vi "AI0.vi"(8 "error in (no error)":errorcluster caption="错误输入（无错误）") -> (0 "error out":errorcluster caption="错误输出", 3 "Ai0波形":waveform(dbl)(graph))   [LabVIEW 2016]
uses:
  <vilib>/DAQmx/read.llb/DAQmx Read (Analog Wfm 1Chan NSamp).vi
  <vilib>/DAQmx/create/channels.llb/DAQmx Create Channel (AI-Voltage-Basic).vi
  <vilib>/DAQmx/configure/timing.llb/DAQmx Timing (Sample Clock).vi
  <vilib>/DAQmx/miscellaneous.llb/DAQmx Fill In Error Info.vi
  <vilib>/DAQmx/create/channels.llb/DAQmx Create Channel (AO-Voltage-Basic).vi
  <vilib>/DAQmx/configure/trigger.llb/DAQmx Start Trigger (None).vi
  <vilib>/DAQmx/write.llb/DAQmx Write (Analog Wfm 1Chan NSamp).vi
  <vilib>/measure/NI_MABase.lvlib
  <resource>/objmgr/daqmx.rc
panel:
  out "输出波形":waveform(dbl)(graph)
  in  "输出数组":cluster{"波形类型":u16, "幅值":dbl, "频率":dbl}[](array[cluster]) {"频率" format="%0.2p"; "幅值" format="%0.2p"; "波形类型" items=["正弦波", "三角波", "方波", "锯齿波"]}
  in  "采样数":i32=100
  out "Ai0波形 2":waveform(dbl)(graph)
  out "电阻":dbl
  in  "停止":bool
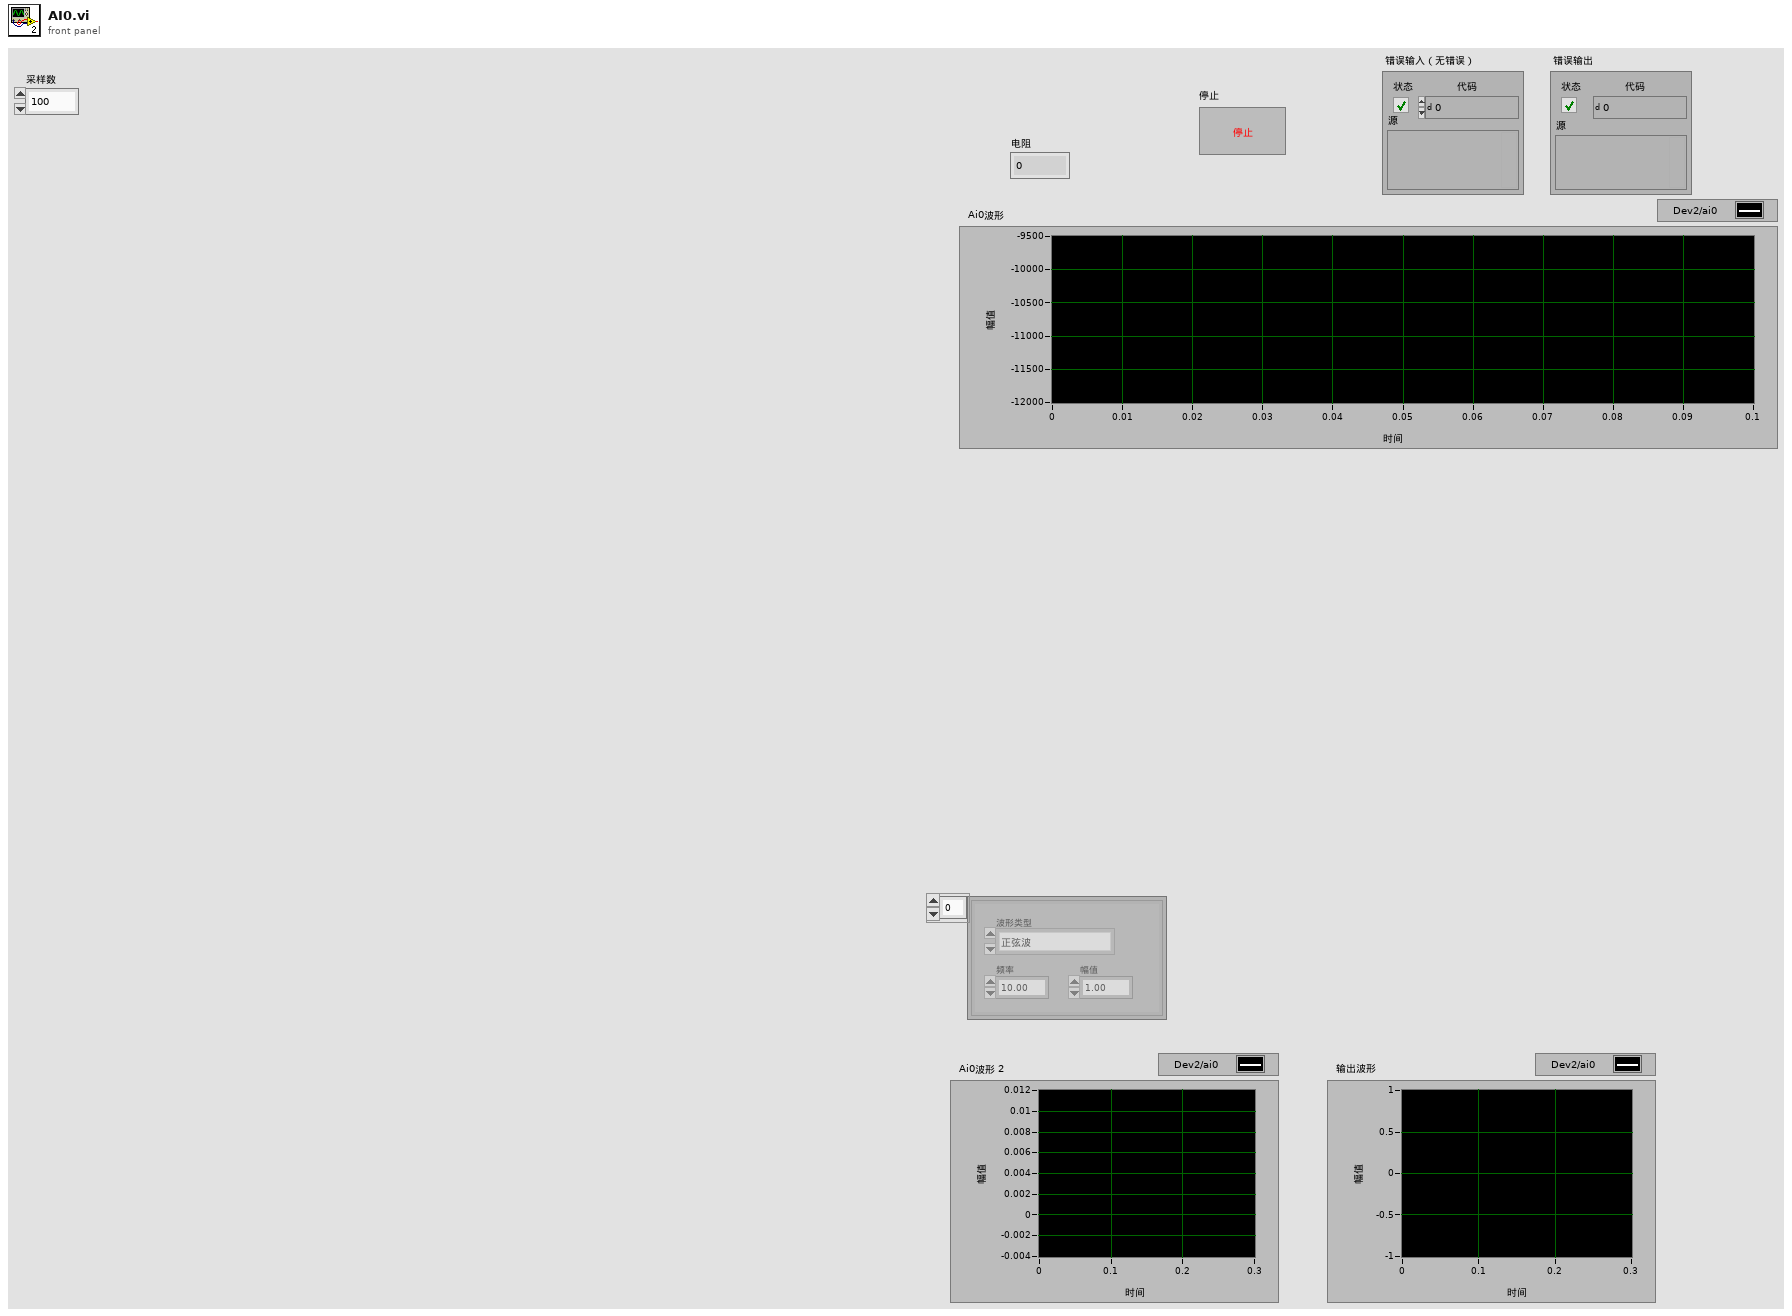
[diagram p1: front panel]
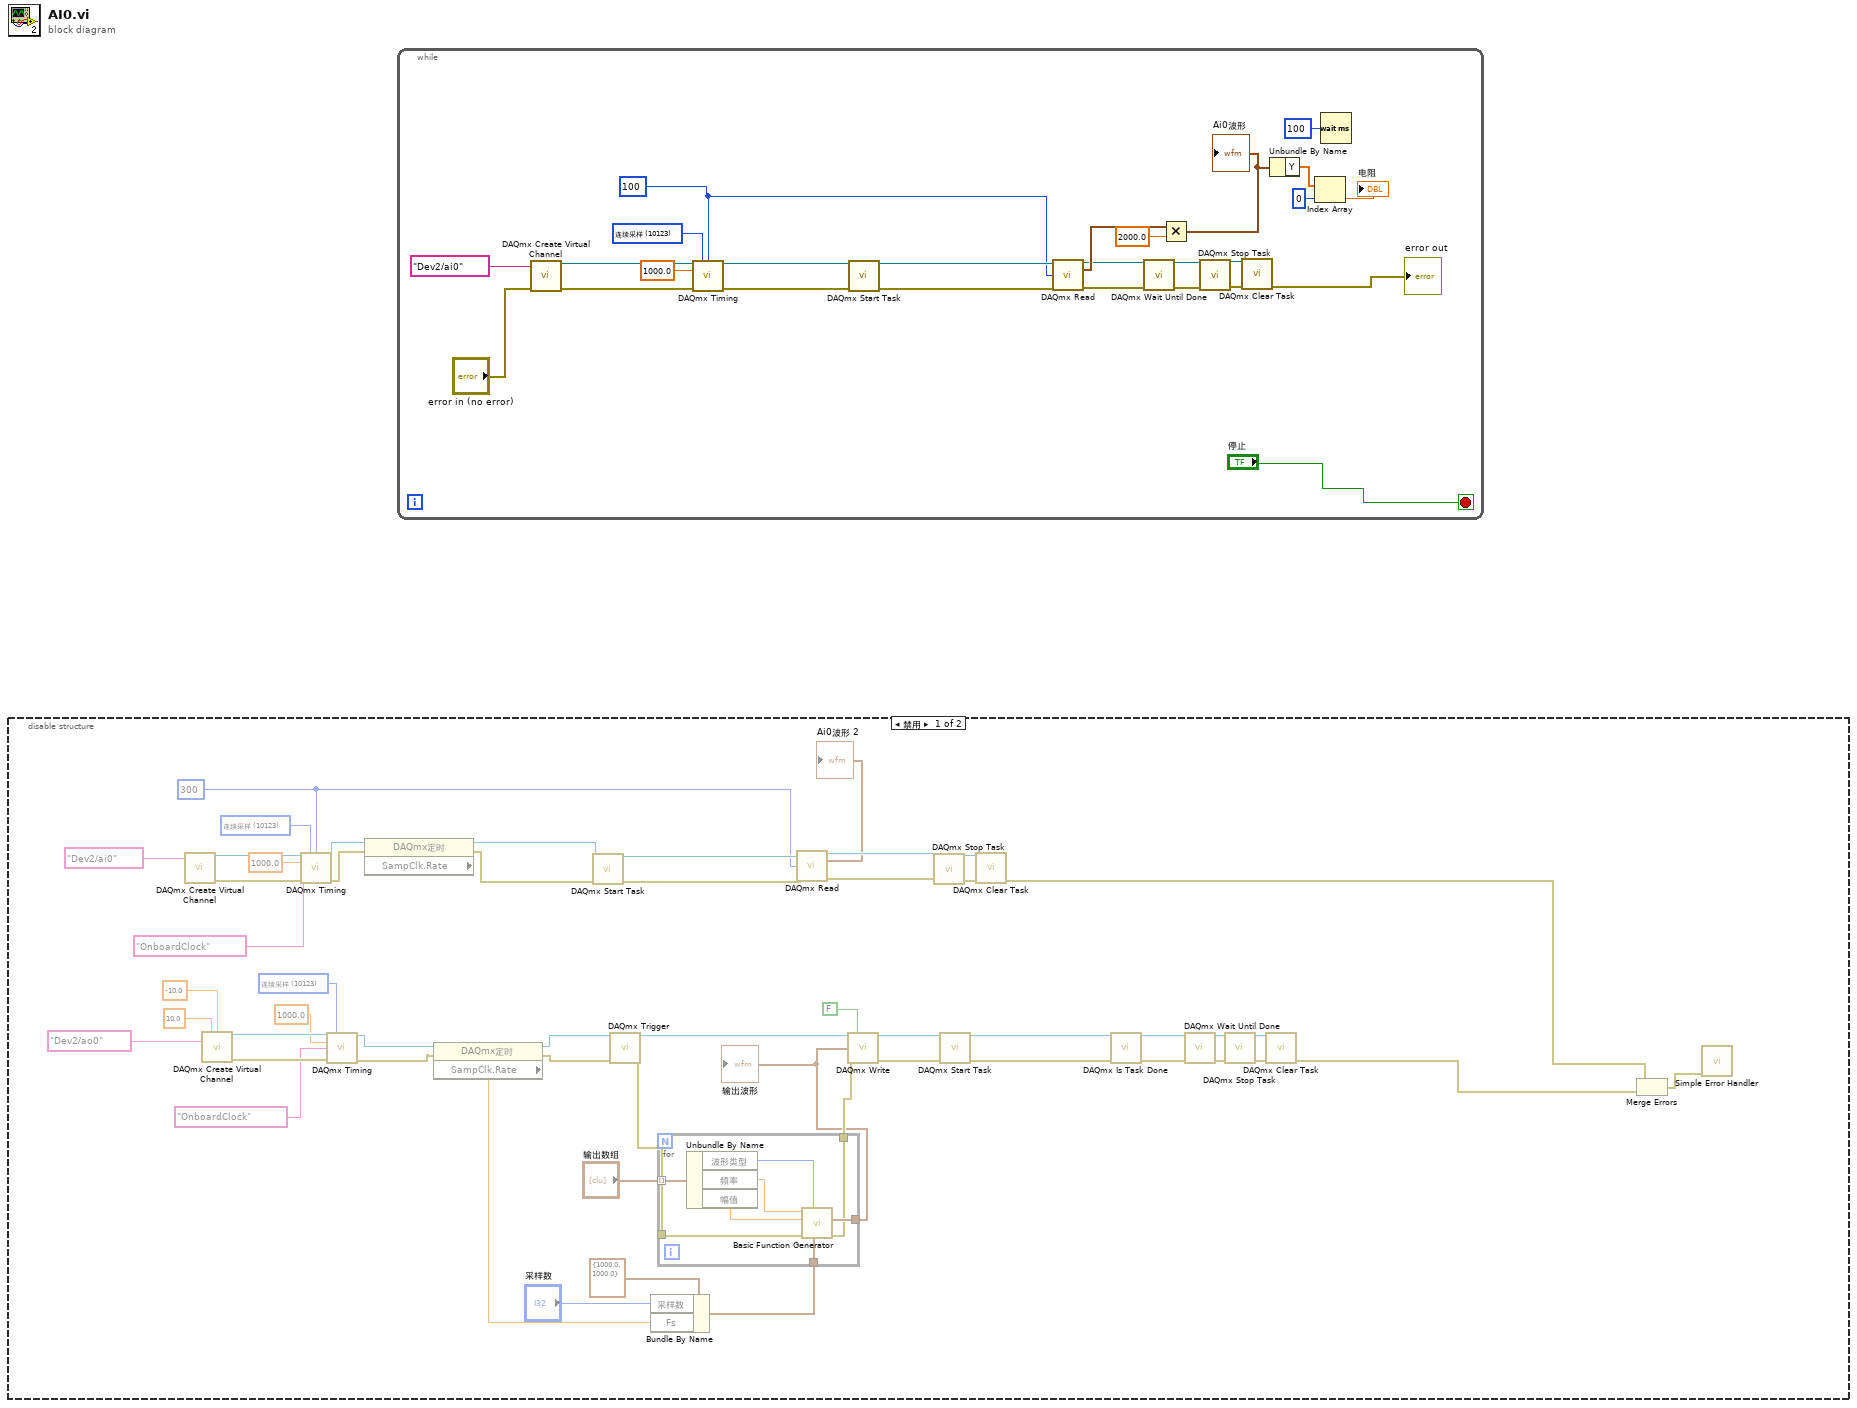
[diagram p0: block diagram]
diagram:
  n1 = disable-structure shown="禁用" {
    frame Disabled {
      w6 = 300
      w34 = 10123 items=["有限采样"=10178, "连续采样"=10123, "硬件定时单点"=12522] ("sample mode")
      w48 = 10123 items=["有限采样"=10178, "连续采样"=10123, "硬件定时单点"=12522] ("sample mode")
      n2 = call-poly <vilib>:"DAQmx Create Virtual Channel.vi"("physical channels"=tag "Dev2/ai0") -> ("task out"=w49:refnum<k21>, "error out"=w50:errorcluster)  [unwired: 13 in]
      n3 = call-poly <vilib>:"DAQmx Create Virtual Channel.vi"("maximum value"=10.0, "minimum value"=-10.0, "physical channels"=tag "Dev2/ao0") -> ("task out"=w36:refnum<k21>, "error out"=w35:errorcluster)  [unwired: 11 in]
      n4 = call-poly <vilib>:"DAQmx Timing.vi"("task/channels in"=w49, "sample mode"=w48, "samples per channel"=w6, "rate"=1000.0, "source"=tag "OnboardClock", "error in"=w50) -> ("task out"=w5:refnum<k21>, "error out"=w4:errorcluster)  [unwired: 8 in]
      n5 = call-poly <vilib>:"DAQmx Timing.vi"("task/channels in"=w36, "sample mode"=w34, "rate"=1000.0, "source"=tag "OnboardClock", "error in"=w35) -> ("task out"=w23:refnum<k21>, "error out"=w21:errorcluster)  [unwired: 9 in]
      n6 = property class="DAQmx定时" props=["SampClk.Rate"](reference=w5, error in=w4) -> (reference out=w3:refnum<k21>, error out=w2:errorcluster)  [unwired: 1 out]
      n7 = property class="DAQmx定时"(reference=w23, error in=w21) -> (reference out=w22:refnum<k21>, error out=w20:errorcluster, "SampClk.Rate"=w19:dbl)
      n8 = call <vilib>:"DAQmx Start Task.vi"("task/channels in"=w3, "error in"=w2) -> ("task out"=w43:refnum<k21>, "error out"=w42:errorcluster)  [unwired: 12 in]
      n9 = call-poly <vilib>:"DAQmx Trigger.vi"("task/channels in"=w22, "error in"=w20) -> ("task out"=w30:refnum<k21>, "error out"=w26:errorcluster)  [unwired: 12 in]
      n10 = Bundle By Name(cluster=cluster{"Fs":dbl, "采样数":dbl} {"Fs"=1000.0, "采样数"=1000.0} ("采样信息"), "采样数"="采样数", "Fs"=w19) -> (w17:cluster{"Fs":dbl, "采样数":dbl})
      n11 = for {
        tunnel: "输出数组" -> [w58] mode=indexing
        tunnel: [w61] -> w24
        tunnel: w26 -> [w60]
        tunnel: [w59] -> w25
        tunnel: w17 -> [w54]
        n12 = Unbundle By Name(w58) -> ("波形类型"=w57:u16, "频率"=w56:dbl, "幅值"=w55:dbl)
        n13 = call <vilib>:"Basic Function Generator.vi"("sampling info"=w54, "signal type"=w57, "error in (no error)"=w60, "amplitude"=w55, "frequency"=w56) -> ("error out"=w59:errorcluster, "signal out"=w61:waveform(dbl))  [unwired: 4 in, 1 out]
      }
      "输出波形" <- w24
      n14 = call-poly <vilib>:"DAQmx Read.vi"("task/channels in"=w43, "number of samples per channel"=w6, "error in"=w42) -> ("task out"=w41:refnum<k21>, "data"=→"Ai0波形 2":waveform(dbl), "error out"=w40:errorcluster)  [unwired: 10 in]
      n15 = call-poly <vilib>:"DAQmx Write.vi"("task/channels in"=w30, "auto start"=FALSE, "data"=w24, "error in"=w25) -> ("task out"=w29:refnum<k21>, "error out"=w28:errorcluster)  [unwired: 9 in, 1 out]
      n16 = call <vilib>:"DAQmx Stop Task.vi"("task/channels in"=w41, "error in"=w40) -> ("task out"=w53:refnum<k21>, "error out"=w52:errorcluster)  [unwired: 12 in]
      n17 = call <vilib>:"DAQmx Start Task.vi"("task/channels in"=w29, "error in"=w28) -> ("task out"=w45:refnum<k21>, "error out"=w44:errorcluster)  [unwired: 12 in]
      n18 = call <vilib>:"DAQmx Clear Task.vi"("task in"=w53, "error in"=w52) -> ("error out"=w38:errorcluster)  [unwired: 13 in]
      n19 = call <vilib>:"DAQmx Is Task Done.vi"("task/channels in"=w45, "error in"=w44) -> ("task out"=w10:refnum<k21>, "error out"=w9:errorcluster)  [unwired: 11 in, 1 out]
      n20 = call <vilib>:"DAQmx Wait Until Done.vi"("task/channels in"=w10, "error in"=w9) -> ("task out"=w13:refnum<k21>, "error out"=w12:errorcluster)  [unwired: 12 in]
      n21 = call <vilib>:"DAQmx Stop Task.vi"("task/channels in"=w13, "error in"=w12) -> ("task out"=w14:refnum<k21>, "error out"=w11:errorcluster)  [unwired: 12 in]
      n22 = call <vilib>:"DAQmx Clear Task.vi"("task in"=w14, "error in"=w11) -> ("error out"=w39:errorcluster)  [unwired: 13 in]
      n23 = Merge Errors(w38, w39) -> (w37:errorcluster)
      n24 = call <vilib>:"Simple Error Handler.vi"("error in (no error)"=w37) -> ()  [unwired: 4 in, 5 out]
    }
    frame Enabled {
    }
  }
  n25 = while {
    stop <- "停止" stop-if-true
    w78 = 100
    w82 = 10123 items=["有限采样"=10178, "连续采样"=10123, "硬件定时单点"=12522] ("sample mode")
    n26 = call-poly <vilib>:"DAQmx Create Virtual Channel.vi"("physical channels"=tag "Dev2/ai0", "error in"="error in (no error)") -> ("task out"=w83:refnum<k21>, "error out"=w84:errorcluster)  [unwired: 12 in]
    n27 = call-poly <vilib>:"DAQmx Timing.vi"("task/channels in"=w83, "sample mode"=w82, "samples per channel"=w78, "rate"=1000.0, "error in"=w84) -> ("task out"=w75:refnum<k21>, "error out"=w74:errorcluster)  [unwired: 9 in]
    n28 = call <vilib>:"DAQmx Start Task.vi"("task/channels in"=w75, "error in"=w74) -> ("task out"=w80:refnum<k21>, "error out"=w79:errorcluster)  [unwired: 12 in]
    n29 = call-poly <vilib>:"DAQmx Read.vi"("task/channels in"=w80, "number of samples per channel"=w78, "error in"=w79) -> ("task out"=w65:refnum<k21>, "data"=w68:waveform(dbl), "error out"=w63:errorcluster)  [unwired: 10 in]
    n30 = call <vilib>:"DAQmx Wait Until Done.vi"("task/channels in"=w65, "error in"=w63) -> ("task out"=w64:refnum<k21>, "error out"=w62:errorcluster)  [unwired: 12 in]
    n31 = Multiply(x=w68, y=2000.0) -> (x*y=w66:waveform(dbl))
    "Ai0波形" <- w66
    n32 = call <vilib>:"DAQmx Stop Task.vi"("task/channels in"=w64, "error in"=w62) -> ("task out"=w87:refnum<k21>, "error out"=w86:errorcluster)  [unwired: 12 in]
    n33 = call <vilib>:"DAQmx Clear Task.vi"("task in"=w87, "error in"=w86) -> ("error out"=→"error out":errorcluster)  [unwired: 13 in]
    n34 = Unbundle By Name(w66) -> ("Y"=w72:dbl[])
    n35 = Index Array(array=w72, index=0 ("索引")) -> (element=→"电阻":dbl)
    n36 = Wait (ms)(milliseconds to wait=u32 100 ("等待时间（毫秒）")) -> ()  [unwired: 1 out]
  }
